vi "AlliGator Load ROIs, Select one ROI (& Convert to Pixel ROIs) Script.vi"(6 "Convert to single Pixel ROIs":bool, 8 "Error In":errorcluster, 9 "ROI ID":i32, 11 "ROI File":path) -> (0 "Error Out":errorcluster, 3 "Load & Convert ID'ed ROI to pixel ROIs":T1[](array[typedef]))   [LabVIEW 2021, in "AlliGator Scripts.lvlib"]
doc: "Script loading the selected ROI from a multi-ROIs file,\n\nThis requires a number of subsequent steps that are queued by this script."
uses:
  AlliGator Scripts.lvlib
  AlliGator Q Element.ctl
  AlliGator Q Event.ctl
  AlliGator ROI Manager Actions.ctl
  AlliGator Action Engine.lvlib
  AlliGator ROIs.lvlib
panel:
  # "see the AlliGator License on the block diagram (Ctrl+E or Window:Show Block Diagram)"
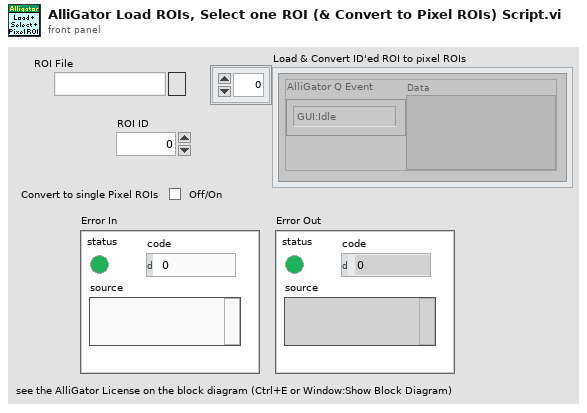
[diagram p1: front panel]
types:
  T1 = typedef "AlliGator Action Engine.lvlib/AlliGator Q Element.ctl" = cluster{"AlliGator Q Event":T2, "Data":variant}
  T2 = typedef "AlliGator Action Engine.lvlib/AlliGator Q Event.ctl" = enum16{"---- Files ----", "Files:Set Batch Export Files To Save", "Files:Set Dataset Loading & Pre-processing Options", "Files:Check #Frames in Dataset", "Files:Increment Frame Index", "Files:Open Mask Image", "Files:Open White Light Image", "Files:Open Single Dataset", "Files:New Folder of Folders Selected", "Files:Load File (all Types)_Scriptable", "Files:Move Flattened Series to Folders Series", "Files:Select Folder", "Files:Load FLI Dataset", "Files:Load Swiss SPAD 1 Dataset", "Files:Load Swiss SPAD 2 Dataset", "Files:Load .sdt FLI Dataset", "Files:Load .ptu FLI Dataset", "Files:Load .bin FLI Dataset", "Files:Load Single Gate Image Folder", "Files:Load I/m/phi Dataset (deprecated)", "Files:Load Single Image", "Files:Subtract Background File", "Files:Export FLI Dataset", "Files:Load HDF5 FLI Dataset", "Files:Set Destination File Path", "Files:Save Mask Image", "Files:Batch Conversion", "Files:New Folder Selected", "Files:Close FLI Dataset", "Files:Close FLI Dataset Series", "Files:Close White Light Image", "Files:Close Mask Image", "---- FLI Dataset ----", "FLI Dataset:Channel Arithmetic", "FLI Dataset:Export Average Lifetime Map as ASCII", "FLI Dataset:Export User-Defined Quantity Map as ASCII", "FLI Dataset:Python Function FLI Dataset Event", "FLI Dataset:ROI Analysis", "FLI Dataset:Tilted Logistic Square Gated IRF Characteristics Map", "FLI Dataset:Logistic Square Gated IRF Characteristics Map", "FLI Dataset:Square Gated IRF Characteristics Map", "FLI Dataset:Multi-ROI Single-Pixel Phasor Analysis", "FLI Dataset:Multi-ROI Single-Pixel NLSF Analysis", "FLI Dataset:All ROIs IRF Extraction", "FLI Dataset:All ROIs Decay Fit Non-Interactive (Fast + Individual IRF)", "FLI Dataset:All ROIs Phasor Analysis", "FLI Dataset:All ROIs Decay Fit", "FLI Dataset:Fluorescence Decay Statistics", "FLI Dataset:Update Decay Statistics Graph", "FLI Dataset:Get Decay from ROI", "FLI Dataset:All ROIs Average Lifetimes", "---- FLI Dataset Series ----", "FLI Dataset Series:Sum All Datasets in Series", "FLI Dataset Series:Add Dataset to Accumulated Dataset", "FLI Dataset Series:Display Accumulated Dataset", "FLI Dataset Series:Clear Dataset Series Sum", "FLI Dataset Series:Time-Series Analysis (NLSF)", "FLI Dataset Series:Time-Series Analysis (Phasor)", "---- Image ----", "Image:Update Image Profile Plots", "Image:Image Histogram Cursor Move", "Image:Image Histogram", "Image:Image Contrast", "Image:Set Image Histogram Cursor Move Flag", "Image:Clear Image Overlay", "Image:Use ROI as Search Area", "Image:Set ROI Diameter", "Image:Save Image Data as TIFF", "Image:Save Displayed Image with Overlay", "Image:Save Image Overlay Only", "Image:Save Image as Hot Pixel Mask", "Image:Change Source Image Color Palette", "Image:Copy Image to Clipboard", "Image:Source Image ROI Selection", "Image:Delete All ROIs", "Image:Delete All Unselected ROIs", "Image:Delete ROI", "Image:Merge All ROIs", "Image:Store ROI", "Image:Source Image ROI Storage", "Image:Export ROI Description to Notebook", "Image:Save ROI", "Image:Load ROI", "Image:Paste ROI Definition", "Image:Clear ROI", "Image:Identify ROIs in Mask Image", "Image:Create Complementary ROI", "Image:Create Contour ROI", "Image:Create ROI(s) from Pixels with Peak above Min_Scriptable", "Image:Create ROI(s) from Pixels with Intensity above Min_Scriptable", "Image:Compute ROI Statistics", "Image:Delete ROI(s) based on ROI Characteristics", "Image:Create ROI Grid", "Image:ROI to Individual Pixel ROIs", "Image:Python Function Source Image Event", "Image:Show Phasor Calibration Map ROI Centers", "Image:Convert ROI to Mask Image", "Image:Mouse Move", "Image:Mouse Up", "Image:Set Source Image Mouse Move Flag", "Image:Add Scale Bar Overlay", "Image:Delete Existing ROIs Option", "---- Decay ----", "Decay:Clear IRF/Reference Plot", "Decay:Clear Local IRFs", "Decay:Add Decay to Graph", "Decay:Smoothen Plot", "Decay:Smoothen Plot Tail", "Decay:Average Selected Plots", "Decay:Extract IRF", "Decay:Optimal IRF Extraction", "Decay:Threshold IRF", "Decay:Fit to Model IRF", "Decay:Fit IRF to Square Gate", "Decay:Fit IRF to Logistic Square Gate", "Decay:Fit IRF to Tilted Logistic Square Gate", "Decay:Create Bounding Cursors Set", "Decay:Export Bounding Cursors Definition to Notebook", "Decay:Denoise Plot", "Decay:Compute Cumulative Function", "Decay:Use as Reference Decay", "Decay:Show Reference Decay/IRF", "Decay:Extrapolate Decay", "Decay:Create Head & Tail Bounding Cursors", "Decay:Store Cursor-defined Head & Tail Fractions", "Decay:Rebin Plot", "Decay:1-Normalize Decay", "Decay:[0-1]-Normalize Plot", "Decay:Straighten Decay", "Decay:Shift Decay", "Decay:Fold Decay", "Decay:Fit Decay", "Decay:Global Fit of Selected Decays", "Decay:Post Global Fit Script", "Decay:Add Global Fit Parameters to Graph", "Decay:Add Decay Parameter(s) to Plot (Graph)", "Decay:Export Decay to Phasor Graph", "Decay:Plot Decay Shifts", "Decay:Compute Average Lifetime", "Decay:Plot Convolution", "Decay:Graph Tip Strip Update", "---- Decay Statistics ----", "Decay Statistics:Tip Strip Update", "---- Intensity Time Trace ----", "Intensity Time Trace:Use File Timestamp", "Intensity Time Trace:Load Intensity Corrections File", "Intensity Time Trace:Clear Intensity Corrections File", "Intensity Time Trace:Tip Strip Update", "---- Phasor Plot ----", "Phasor Plot:Build Phasor Plot", "Phasor Plot:Change Phasor Plot Color Palette", "Phasor Plot:Adjust Phasor Plot Display Range", "Phasor Plot:Highlight Image ROI in Phasor Plot", "Phasor Plot:Save Phasor Plot Image with Overlay", "Phasor Plot:Export Complex Phasor Map", "Phasor Plot:Export Phasor Ratio Map", "Phasor Plot:Export Average Lifetime Map", "Phasor Plot:Compute Phase Lifetime Histogram", "Phasor Plot:Compute Phasor Ratio Histogram", "Phasor Plot:Compute Phase Lifetime vs Intensity Scatter Plot", "Phasor Plot:Weber 2-Component Decomposition", "Phasor Plot:Update Phasor Color Map Vertices", "Phasor Plot:Clear Phasor Overlay", "Phasor Plot:Use Segment Extremities as References", "Phasor Plot:Use UC/Segment Intersections as References", "Phasor Plot:Use UC/Principal Axis Intersections as References", "Phasor Plot:Use UC/Linear Fit Intersections as References", "Phasor Plot:Update Phasor Plot Reference", "Phasor Plot:Show Local Phasor Info in Phasor Plot", "Phasor Plot:Update Phasor Plot State", "Phasor Plot:Phasor Plot ROI Storage", "Phasor Plot:Phasor Plot ROI Selection", "Phasor Plot:Python Function Phasor Plot Event", "Phasor Plot:Overlay Phasor ROI, Ratio or Map in Source Image", "Phasor Plot:Compute Decay of Selected Phasors", "Phasor Plot:Phasor at Image Pixel", "Phasor Plot:Mouse Move", "Phasor Plot:Mouse Up", "Phasor Plot:Display Range Mouse Move", "Phasor Plot:Set Mouse Move Flag", "---- Phasor Graph ----", "Phasor Graph:Calibrated Phasor Map Series", "Phasor Graph:Whole Image Phasor Scatter Plot (Todo)", "Phasor Graph:Get Phasor Value", "Phasor Graph:Create New Phasor Plot Dialog", "Phasor Graph:Update Last Phasor Value", "Phasor Graph:Update Phasor (m, phi)", "Phasor Graph:Remove Single Phasor from Plot", "Phasor Graph:Add Single Phasor to Plot", "Phasor Graph:Remove Phasor Plot", "Phasor Graph:Remove Selected Phasor Plots", "Phasor Graph:Clear Phasor Data", "Phasor Graph:Clear Phasor Graph", "Phasor Graph:Cursor Move", "Phasor Graph:Draw Cursor Connecting Line", "Phasor Graph:Clear Cursor Connecting Line", "Phasor Graph:Find UC Intersection", "Phasor Graph:Use UC/Cursor-Defined Line Intersections", "Phasor Graph:Use Selected Plots Fitted Line/UC Intersections", "Phasor Graph:Use Selected Plots Principal Axis/UC Intersections", "Phasor Graph:Show Single Phasor", "Phasor Graph:Save Single Phasor Plot", "Phasor Graph:Save All Phasor Plots", "Phasor Graph:Load Phasor Plot(s)", "Phasor Graph:Phasor Multiplication", "Phasor Graph:Compute Average Phasor", "Phasor Graph:Compute Multiple Average Phasors (Selected Plots)", "Phasor Graph:Export Single Phasor Plot Phase Lifetimes", "Phasor Graph:Phase Lifetime Trajectory", "Phasor Graph:Phase Lifetime vs Intensity Scatter Plot (deprecated)", "Phasor Graph:Parameter 2 vs Parameter 1 Scatter Plot", "Phasor Graph:Use Cursor n Location", "Phasor Graph:Set Reference n to Current Phase Lifetime Value", "Phasor Graph:Set Reference n to Lifetime Value", "Phasor Graph:Set Cursor n Location", "Phasor Graph:Save Phasor Graph Image", "Phasor Graph:Update SEPL Plot", "Phasor Graph:Export Single Phasor Plot Data", "Phasor Graph:Export Selected Phasor Plots Data", "Phasor Graph:Python Function Phasor Graph Event", "Phasor Graph:Tip Strip Update", "---- Calibration ----", "Calibration:Set Calibration Type", "Calibration:Load/Save Phasor Calibration", "Calibration:Load/Save Phasor Calibration Series", "Calibration:Load/Save Phasor Calibration Map", "Calibration:Use as Calibration", "Calibration:Compute Optimal Calibration from Phasor References", "Calibration:Clear Phasor Calibration", "Calibration:Single Phasor Calibration Information", "Calibration:Use as Calibration Series", "Calibration:Use as Calibration Map", "Calibration:Clear Calibration Series", "Calibration:Phasor Calibration Series Information", "Calibration:Clear Calibration Map", "Calibration:Phasor Calibration Map Information", "Calibration:Apply Phasor Calibration", "Calibration:Update Single Plot Calibration", "Calibration:Update Multiple Plots Calibration", "Calibration:Clear Single Plot Calibration", "Calibration:Clear All Plots Calibrations", "Calibration:Clear Plot(s) Calibration(s)?", "Calibration:Phasor Calibration Maps (# Gates Series)", "---- Phasor Ratio ----", "Phasor Ratio:Clear Reference n", "Phasor Ratio:Toggle Selected Plot(s)  Lock to Reference 1", "Phasor Ratio:Use as Reference n", "Phasor Ratio:Send Reference n to Notebook", "Phasor Ratio:Toggle Selected Plot(s)  Lock to Reference 2", "Phasor Ratio:Compute Phasor Ratio at Mouse Location", "Phasor Ratio:Compute Phasor Plot's Average Phasor Ratio", "Phasor Ratio:Compute Time-Series Phasor Ratios", "Phasor Ratio:Fit Line to Phasor Ratio Plot", "Phasor Ratio:Save References", "Phasor Ratio:Load References", "Phasor Ratio:Update Phasor Reference 1", "Phasor Ratio:Update Phasor Reference 2", "Phasor Ratio:Move Cursor n to Reference n", "Phasor Ratio:Use as Phasor Reference 1 Lifetime", "Phasor Ratio:Use as Phasor Reference 2 Lifetime", "Phasor Ratio:Export Phasor Ratio Map as ASCII", "Phasor Ratio:Tip Strip Update", "---- Lifetime & Other Parameters Graph ----", "Lifetime:Tip Strip Update", "---- Decay Fit Parameter Map ----", "Decay Fit Parameter Map:Export ROI NLSF Data as ASCII", "Decay Fit Parameter Map:Set Decay Fit  Parameter Map Selection", "Decay Fit Parameter Map:Build Decay Fit Parameter Map", "Decay Fit Parameter Map:Change Decay Fit Parameter Map Color Palette", "Decay Fit Parameter Map:Export Decay Fit Parameter Map Data as ASCII", "Decay Fit Parameter Map:Export All Decay Fit Parameter Maps Data as ASCII", "Decay Fit Parameter Map:Send Map Data to Lifetime Graph", "Decay Fit Parameter Map:Save Decay Fit Parameter Map Image", "Decay Fit Parameter Map:Save-Load IRFs & Fit Data", "Decay Fit Parameter Map:Update Local Decay Plots", "Decay Fit Parameter Map:Python Function Decay Fit Parameters Map Event", "Decay Fit Parameter Map:Overlay Decay Fit Parameter Map in Source Image", "Decay Fit Parameter Map:Plot Map Data vs Intensity", "Decay Fit Parameter Map:Mouse Up", "Decay Fit Parameter Map:Display Range Mouse Move", "---- Generic Graph ----", "Generic Graph:Generic XY Graph Event", "Generic Graph:Python Function XY Graph Event", "Generic Graph:New Plot", "Generic Graph:Save Plot", "Generic Graph:XY Plot Histogram", "Generic Graph:Set XY Graph Plot Name", "Generic Graph:Set Last Cursor Style", "Generic Graph:Tip Strip Update", "---- GUI ----", "GUI:Start Script", "GUI:Type of Displayed Image Changed", "GUI:Gate Image Slide Changed", "GUI:Show Busy Icon", "GUI:Show Busy Icon & Abort Button", "GUI:Hide Busy Icon", "GUI:Hide Busy Icon & Abort Button", "GUI:Abort", "GUI:End Script", "GUI:Start Timing", "GUI:End Timing", "GUI:Set State Indicator", "GUI:Send Parameters JSON Strings to Clipboard", "GUI:Set Gate Step", "GUI:Idle", "GUI:Initialization", "GUI:Quit", "GUI:Increment Dataset Index", "GUI:Set Dataset Index to -1", "GUI:Time Series Slider Moved", "GUI:Time Series Slider Changed", "GUI:Toggle Playback or Loop", "GUI:Playback Script", "GUI:Set Phasor Frequency", "GUI:Open Window", "GUI:Start Test Script", "GUI:End Test Script", "DEBUG"}
  T3 = typedef "AlliGator ROIs.lvlib/AlliGator ROI Manager Actions.ctl" = enum16{"Undefined", "Delete Current ROI", "Delete All Unselected ROIs", "Delete Multiple ROIs", "Delete All ROIs", "Swap ROIs", "Insert ROI", "Update Current ROI Descriptor", "Rename Current ROI", "Store New ROI", "Store Multiple ROIs", "Select Next ROI", "Select Previous ROI", "Find Selected ROI", "Show All ROIs", "Update ROI Manager Window", "Merge All ROIs", "Unmerge ROI", "Set Selected ROI by ID"}
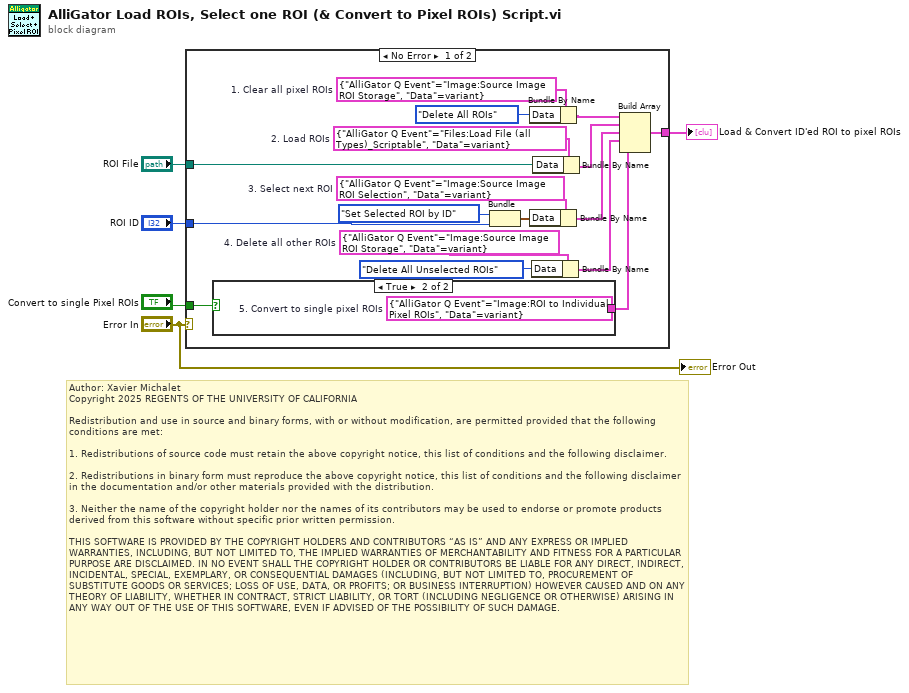
[diagram p0: block diagram]
diagram:
  # "Author: Xavier Michalet\nCopyright 2025 REGENTS OF THE UNIVERSITY OF CALIFORNIA\n\nRedistribution and use in source and binary forms, with or without modification, are permitted provided that the following conditions are met:\n\n1. Redistributions of source code must retain the above copyright notice, this list of conditions and the following disclaimer.\n\n2. Redistributions in binary form must reproduce the above copyright notice, this list of conditions and the following disclaimer in the documentation and/or other materials provided with the distribution.\n\n3. Neither the name of the copyright holder nor the names of its contributors may be used to endorse or promote products derived from this software without specific prior written permission.\n\nTHIS SOFTWARE IS PROVIDED BY THE COPYRIGHT HOLDERS AND CONTRIBUTORS “AS IS” AND ANY EXPRESS OR IMPLIED WARRANTIES, INCLUDING, BUT NOT LIMITED TO, THE IMPLIED WARRANTIES OF MERCHANTABILITY AND FITNESS FOR A PARTICULAR PURPOSE ARE DISCLAIMED. IN NO EVENT SHALL THE COPYRIGHT HOLDER OR CONTRIBUTORS BE LIABLE FOR ANY DIRECT, INDIRECT, INCIDENTAL, SPECIAL, EXEMPLARY, OR CONSEQUENTIAL DAMAGES (INCLUDING, BUT NOT LIMITED TO, PROCUREMENT OF SUBSTITUTE GOODS OR SERVICES; LOSS OF USE, DATA, OR PROFITS; OR BUSINESS INTERRUPTION) HOWEVER CAUSED AND ON ANY THEORY OF LIABILITY, WHETHER IN CONTRACT, STRICT LIABILITY, OR TORT (INCLUDING NEGLIGENCE OR OTHERWISE) ARISING IN ANY WAY OUT OF THE USE OF THIS SOFTWARE, EVEN IF ADVISED OF THE POSSIBILITY OF SUCH DAMAGE."
  n1 = case shown="No Error" "Error In" {
    tunnel: "ROI ID" -> [w21 _]
    tunnel: "ROI File" -> [w17 _]
    tunnel: [w7 _] -> w3
    tunnel: "Convert to single Pixel ROIs" -> [w6 _]
    frame No Error {
      w16 = T1 {"AlliGator Q Event"=enum."Files:Load File (all Types)_Scriptable", "Data"=variant}  # 2. Load ROIs
      w18 = T1 {"AlliGator Q Event"=enum."Image:Source Image ROI Storage", "Data"=variant}  # 1. Clear all pixel ROIs
      w14 = T1 {"AlliGator Q Event"=enum."Image:Source Image ROI Storage", "Data"=variant}  # 4. Delete all other ROIs
      w13 = T1 {"AlliGator Q Event"=enum."Image:Source Image ROI Selection", "Data"=variant}  # 3. Select next ROI
      n2 = case shown="True" w6 {
        tunnel: [_ w23] -> w8
        frame False {
        }
        frame True {
          w23 = T1 {"AlliGator Q Event"=enum."Image:ROI to Individual Pixel ROIs", "Data"=variant}  # 5. Convert to single pixel ROIs
        }
      }
      n3 = Bundle("Action"=AlliGator_ROI_Manager_Actions."Set Selected ROI by ID", "ROI ID"=w21) -> (w22:cluster{"Action":T3, "ROI ID":i32})  [unwired: 1 in]
      n4 = Bundle By Name(cluster=w18, "Data"=AlliGator_ROI_Manager_Actions."Delete All ROIs" ("Action")) -> (w12:T1)
      n5 = Bundle By Name(cluster=w13, "Data"=w22) -> (w10:T1)
      n6 = Bundle By Name(cluster=w14, "Data"=AlliGator_ROI_Manager_Actions."Delete All Unselected ROIs" ("Action")) -> (w9:T1)
      n7 = Bundle By Name(cluster=w16, "Data"=w17) -> (w11:T1)
      n8 = Build Array(w12, w11, w10, w9, w8) -> (w7:T1[])
    }
    frame Error {
    }
  }
  "Load & Convert ID'ed ROI to pixel ROIs" <- w3
  "Error Out" <- "Error In"
